vi "SATHdll.vi"(8 "error in (no error)":errorcluster, 11 "SAT Inputs":cluster{"h":dbl, "z":dbl[], "kph":u16}={"h"=0.0, "z"=[0.0, 0.0, 0.0, 0.0, 0.0, 0.0, 0.0, 0.0, 0.0, 0.0, 0.0, 0.0, 0.0, 0.0, 0.0, 0.0, 0.0, 0.0, 0.0, 0.0], "kph"=0} {"kph" items=["0 - Return alll roots along the liquid-vapor line", "1 - Return only liquid VLE root", "2 - Return only vapor VLE roots", "3 - Return liquid SLE root (melting line)", "4 - Return vapor SVE root (sublimation line)"]}) -> (0 "error out":errorcluster, 3 "SAT Outputs":T1={"D"=nan, "e"=nan, "h"=nan, "p"=nan, "s"=nan, "t"=nan, "q"=nan, "Dl"=nan, "Dv"=nan, "x"=[nan, nan, 0.0, 0.0, 0.0, 0.0, 0.0, 0.0, 0.0, 0.0, 0.0, 0.0, 0.0, 0.0, 0.0, 0.0, 0.0, 0.0, 0.0, 0.0], "y"=[nan, nan, 0.0, 0.0, 0.0, 0.0, 0.0, 0.0, 0.0, 0.0, 0.0, 0.0, 0.0, 0.0, 0.0, 0.0, 0.0, 0.0, 0.0, 0.0], "nroot"=0, "k1"=0, "t1"=nan, "p1"=nan, "d1"=nan, "k2"=0, "t2"=nan, "p2"=nan, "d2"=nan, "k3"=0, "t3"=nan, "p3"=nan, "d3"=nan, "ierr"=0, "herr"="", "herr_length"=0})   [LabVIEW 2016]
doc: "subroutine SATHdll(h, z, kph, nroot, k1, t1, p1, d1, k2, t2, p2, d2, ierr, herr, herr_length)\n\nIterate for temperature, pressure, and density given enthalpy along\nthe saturation boundary and the composition.\n\nThe second root is always set as the root in the vapor at temperatures\nbelow the maximum enthalpy on the vapor saturation line. If kph is\nset to 2, and only one root is found in the vapor (this occurs when h<hcrit)\nthe state point will be placed in k2,t2,p2,d2. If kph=0 and this situation\noccurred, the first root (k1,t1,p1,d1) would be in the liquid (k1=1, k2=2).\n\nINPUTS:\n h--molar enthalpy [J/mol]\n z--composition [array of mol frac]\n kph--flag specifying desired root\n 0 = return all roots along the liquid-vapor line\n 1 = return only liquid VLE root\n 2 = return only vapor VLE roots\n 3 = return liquid SLE root (melting line)(only for pure fluids)\n 4 = return vapor SVE root (sublimation line)(only for pure fluids)\n\nOUTPUTS:\n nroot--number of roots. Value is set to one for kph=1,3,4 if ierr=0\n k1--phase of first root (1-liquid, 2-vapor, 3-melt, 4-subl)\n t1--temperature of first root [K]\n p1--pressure of first root [kPa]\n d1--molar density of first root [mol/L]\n k2--phase of second root (1-liquid, 2-vapor, 3-melt, 4-subl)\n t2--temperature of second root [K]\n p2--pressure of second root [kPa]\n d2--molar density of second root [mol/L]\n ierr--error flag: 0 = successful\n 2 = h < hmin\n 4 = h > hmax\n 8 = h > htrp (for subl input)\n 160 = CRITP did not converge\n 161 = SATH did not converge for one root\n 162 = SATH did not converge for both roots\n herr--error string (character*255 variable if ierr<>0)\n herr_length-- length of variable herr (default: 255)"
uses:
  Ctl/SAT_Outputs.ctl
  REFPROP.DLL
panel:
  # "REFPROP-SATHdll.vi"
  # "subroutine SATHdll(h, z, kph, nroot, k1, t1, p1, d1, k2, t2, p2, d2, ierr, herr, herr_length)"
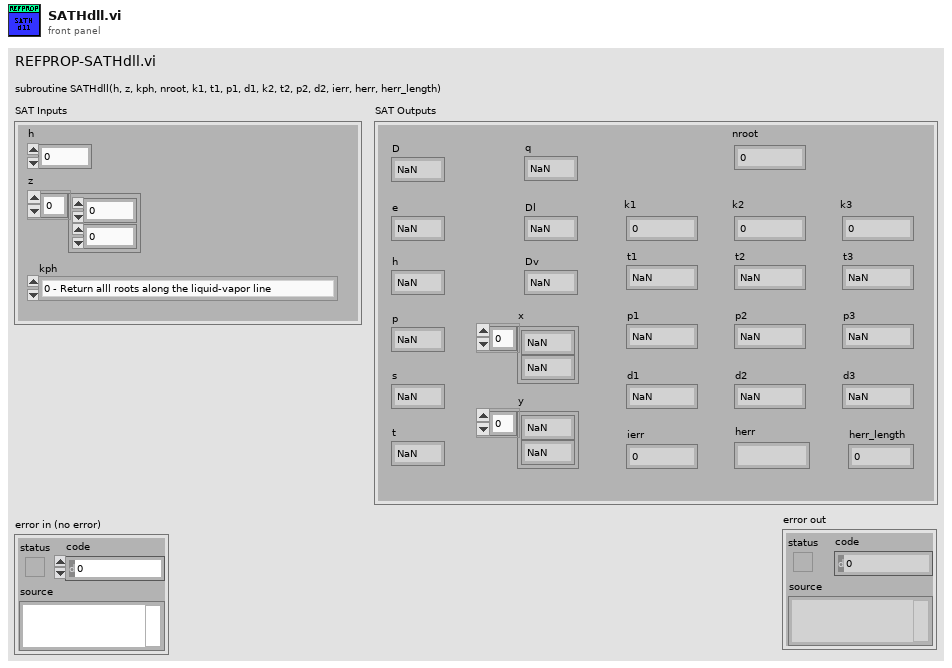
[diagram p1: front panel]
types:
  T1 = typedef "SAT_Outputs.ctl" = cluster{"D":dbl, "e":dbl, "h":dbl, "p":dbl, "s":dbl, "t":dbl, "q":dbl, "Dl":dbl, "Dv":dbl, "x":dbl[], "y":dbl[], "nroot":i32, "k1":i32, "t1":dbl, "p1":dbl, "d1":dbl, "k2":i32, "t2":dbl, "p2":dbl, "d2":dbl, "k3":i32, "t3":dbl, "p3":dbl, "d3":dbl, "ierr":i32, "herr":string, "herr_length":i32}
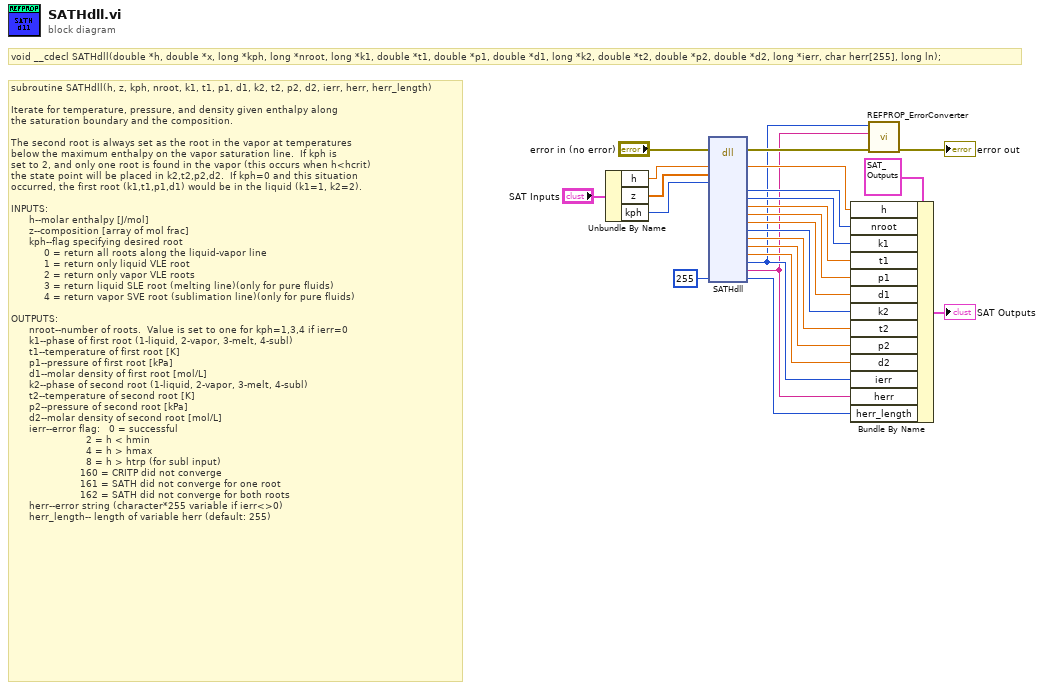
[diagram p0: block diagram]
diagram:
  # "subroutine SATHdll(h, z, kph, nroot, k1, t1, p1, d1, k2, t2, p2, d2, ierr, herr, herr_length)\n\nIterate for temperature, pressure, and density given enthalpy along\nthe saturation boundary and the composition.\n\nThe second root is always set as the root in the vapor at temperatures\nbelow the maximum enthalpy on the vapor saturation line.  If kph is\nset to 2, and only one root is found in the vapor (this occurs when h<hcrit)\nthe state point will be placed in k2,t2,p2,d2.  If kph=0 and this situation\noccurred, the first root (k1,t1,p1,d1) would be in the liquid (k1=1, k2=2).\n\nINPUTS:\n      h--molar enthalpy [J/mol]\n      z--composition [array of mol frac]\n      kph--flag specifying desired root\n           0 = return all roots along the liquid-vapor line\n           1 = return only liquid VLE root\n           2 = return only vapor VLE roots\n           3 = return liquid SLE root (melting line)(only for pure fluids)\n           4 = return vapor SVE root (sublimation line)(only for pure fluids)\n\nOUTPUTS:\n      nroot--number of roots.  Value is set to one for kph=1,3,4 if ierr=0\n      k1--phase of first root (1-liquid, 2-vapor, 3-melt, 4-subl)\n      t1--temperature of first root [K]\n      p1--pressure of first root [kPa]\n      d1--molar density of first root [mol/L]\n      k2--phase of second root (1-liquid, 2-vapor, 3-melt, 4-subl)\n      t2--temperature of second root [K]\n      p2--pressure of second root [kPa]\n      d2--molar density of second root [mol/L]\n      ierr--error flag:   0 = successful\n                         2 = h < hmin\n                         4 = h > hmax\n                         8 = h > htrp (for subl input)\n                       160 = CRITP did not converge\n                       161 = SATH did not converge for one root\n                       162 = SATH did not converge for both roots\n      herr--error string (character*255 variable if ierr<>0)\n      herr_length-- length of variable herr (default: 255)"
  # "void __cdecl SATHdll(double *h, double *x, long *kph, long *nroot, long *k1, double *t1, double *p1, double *d1, long *k2, double *t2, double *p2, double *d2, long *ierr, char herr[255], long ln);"
  n1 = Unbundle By Name("SAT Inputs") -> ("h"=w20:dbl, "z"=w19:dbl[], "kph"=w18:u16)
  n2 = dll-call lib="C:/Program Files (x86)/REFPROP/REFPROP.*" fn="SATHdll"(error in="error in (no error)", "h"=w20, "z"=w19, "kph"=w18, "herr_length"=255 ("ln")) -> (error out=w22:errorcluster, "h"=w13:dbl, "nroot"=w12:i32, "k1"=w11:i32, "t1"=w10:dbl, "p1"=w9:dbl, "d1"=w8:dbl, "k2"=w7:i32, "t2"=w6:dbl, "p2"=w5:dbl, "d2"=w4:dbl, "ierr"=w3:i32, "herr"=w2:string, "herr_length"=w1:i32)  [unwired: 16 in, 1 out]
  n3 = Bundle By Name(cluster=T1 {"D"=nan, "e"=nan, "h"=nan, "p"=nan, "s"=nan, "t"=nan, "q"=0.0, "Dl"=nan, "Dv"=nan, "x"=[nan, nan, 0.0, 0.0, 0.0, 0.0, 0.0, 0.0, 0.0, 0.0, 0.0, 0.0, 0.0, 0.0, 0.0, 0.0, 0.0, 0.0, 0.0, 0.0], "y"=[nan, nan, 0.0, 0.0, 0.0, 0.0, 0.0, 0.0, 0.0, 0.0, 0.0, 0.0, 0.0, 0.0, 0.0, 0.0, 0.0, 0.0, 0.0, 0.0], "nroot"=0, "k1"=0, "t1"=nan, "p1"=nan, "d1"=nan, "k2"=0, "t2"=nan, "p2"=nan, "d2"=nan, "k3"=0, "t3"=nan, "p3"=nan, "d3"=nan, "ierr"=0, "herr"="", "herr_length"=0} ("SAT Outputs"), "h"=w13, "nroot"=w12, "k1"=w11, "t1"=w10, "p1"=w9, "d1"=w8, "k2"=w7, "t2"=w6, "p2"=w5, "d2"=w4, "ierr"=w3, "herr"=w2, "herr_length"=w1) -> (→"SAT Outputs":T1)
  n4 = call "REFPROP_ErrorConverter.vi"("error in (no error)"=w22, "Error Message"=w2, "Error Code"=w3) -> ("error out"=→"error out":errorcluster)  [unwired: 8 in]
